vi "labviewFunc.vi"() -> ()   [LabVIEW 2022 SP3]
uses:
  <vilib>/DAQmx/write.llb/DAQmx Write (Analog DBL 1Chan 1Samp).vi
  <vilib>/DAQmx/read.llb/DAQmx Read (Analog DBL 1Chan 1Samp).vi
  <vilib>/DAQmx/read.llb/DAQmx Read (Counter 1D DBL 1Chan NSamp).vi
  <vilib>/Analysis/baseanly.llb/Mean (DBL).vi
  <vilib>/Utility/error.llb/Trim Whitespace One-Sided.vi
  <vilib>/Utility/file.llb/Read Delimited Spreadsheet (DBL).vi
  <vilib>/Utility/config.llb/Read Key (I32).vi
  <vilib>/Utility/config.llb/Read Key (String).vi
  <vilib>/DAQmx/create/channels.llb/DAQmx Create Channel (CI-Frequency).vi
  <vilib>/DAQmx/configure/timing.llb/DAQmx Timing (Implicit).vi
  <vilib>/DAQmx/create/channels.llb/DAQmx Create Channel (AO-Voltage-Basic).vi
  <vilib>/DAQmx/create/channels.llb/DAQmx Create Channel (AI-Voltage-Basic).vi
  <vilib>/DAQmx/miscellaneous.llb/DAQmx Fill In Error Info.vi
  <resource>/objmgr/daqmx.rc
  <vilib>/Analysis/NI_AALBase.lvlib
  <vilib>/Utility/config.llb/NI_LVConfig.lvlib
  <vilib>/Utility/config.llb/Read Key (Double).vi
panel:
  out "value 4":string
  out "all rows":dbl[](array[numeric])
  out "value 3":string
  out "value 2":string
  out "value":string
  in  "OK Button continue":bool
  in  "OK Button":bool
  out "fvar":variant
  out "ivar":variant
  out "ledVout":dbl[](array[numeric])
  in  "AIChannel":tag
  out "FreqOut":dbl[](array[numeric])
  in  "Delay":u32
  out "error out":errorcluster
  in  "AOChannel":tag
  in  "CounterPFI":tag
  in  "Counter":tag="Dev2/ctr0"
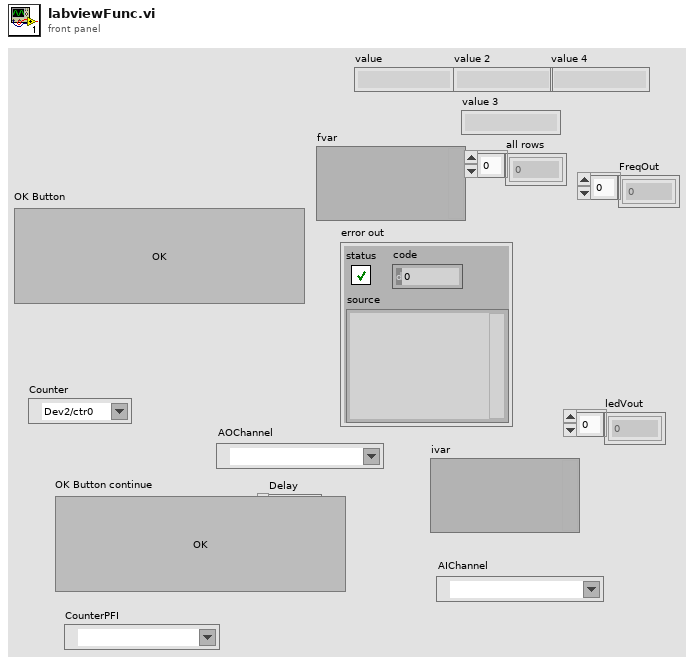
[diagram p1: front panel]
types:
  T1 = enum32{"Invalid", "Standard", "Closed", "Hidden", "Minimized", "Maximized"}
  T2 = typedef "NI_LVConfig.lvlib/Config Data RefNum.ctl" = refnum<k1>
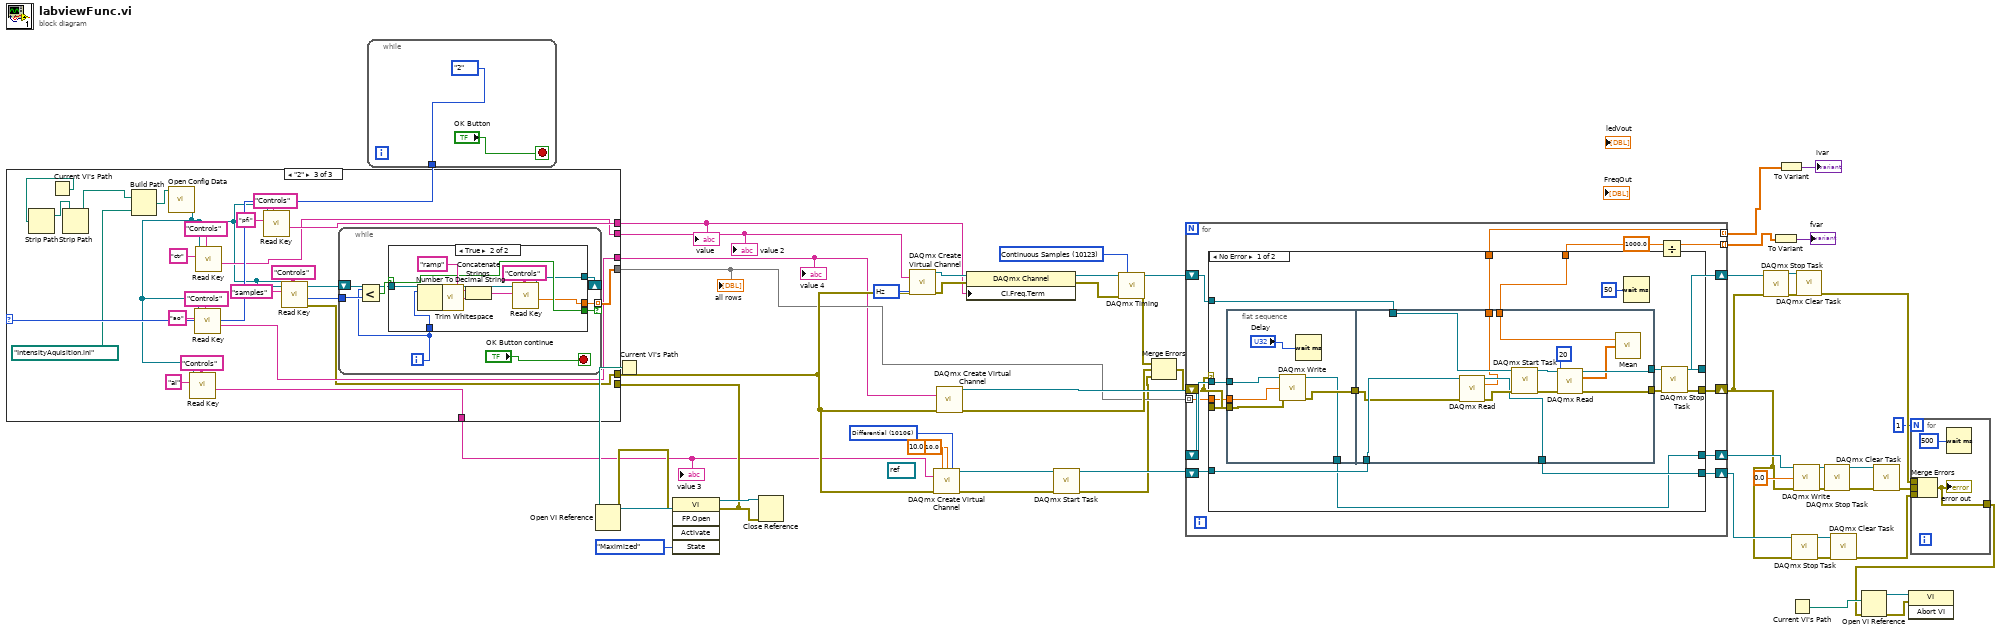
[diagram p0: block diagram]
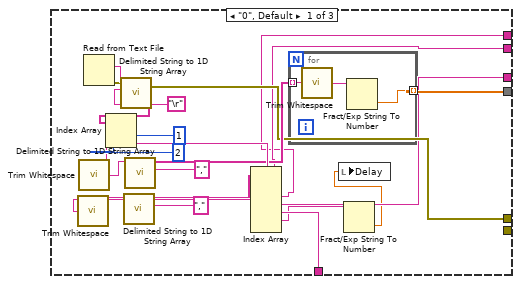
[diagram p2: hidden frame]
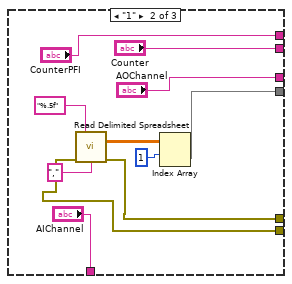
[diagram p3: hidden frame]
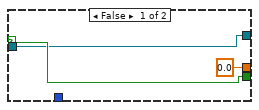
[diagram p4: hidden frame]
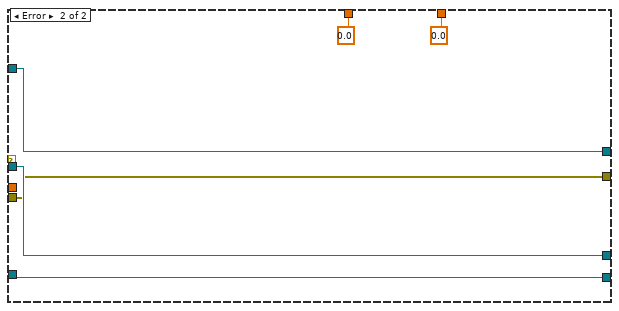
[diagram p5: hidden frame]
diagram:
  w28 = 10106 items=["Default"=-1, "RSE"=10083, "NRSE"=10078, "Differential"=10106, "Pseudodifferential"=12529] ("input terminal configuration")
  (unwired) refnum<k21> refnum ("task out")
  w42 = 10123 items=["Finite Samples"=10178, "Continuous Samples"=10123, "Hardware Timed Single Point"=12522] ("sample mode")
  w45 = 10373 items=["Hz"=10373, "Ticks"=10304, "From Custom Scale"=10065] ("units")
  n1 = while {
    tunnel: [enum16{"0", "1", "2"}."2"] -> w1
    stop <- "OK Button" stop-if-true
  }
  n2 = Current VI's Path() -> (path=w17:path)
  n3 = Open VI Reference(vi path=w17) -> (vi reference=w51:refnum<vi>, error out=w49:errorcluster)  [unwired: 5 in]
  n4 = invoke class="VI" method="FP.Open"(reference=w51, error in=w49, "State"=T1."Maximized") -> (reference out=w48:refnum<vi>, error out=w16:errorcluster)  [unwired: 2 in, 3 out]
  n5 = case shown="\"2\"" w1 {
    tunnel: w16 -> [_ w93 _]
    tunnel: [w67 w91 w101] -> w15
    tunnel: [w68 w89 w109] -> w14
    tunnel: [w65 "Counter" w107] -> w5
    tunnel: [w63 "AOChannel" w106] -> w4
    tunnel: [w62 "AIChannel" w105] -> w3
    tunnel: [w64 "CounterPFI" w108] -> w2
    frame "0", Default {
      n6 = Read from Text File() -> (text=w78:string, error out=w67:errorcluster)  [unwired: 4 in, 2 out]
      n7 = call <vilib>:"Delimited String to 1D String Array.vi"("delimiter"="\r", "delimited string"=w78) -> ("string array"=w77:string[])  [unwired: 9 in]
      n8 = Index Array(array=w77, index #1=1 ("index"), index #2=2 ("index")) -> (element #1=w74:string, element #2=w70:string)
      n9 = call <vilib>:"Trim Whitespace.vi"("string"=w70) -> ("trimmed string"=w59:string)  [unwired: 1 in]
      n10 = call <vilib>:"Trim Whitespace.vi"("string"=w74) -> ("trimmed string"=w73:string)  [unwired: 1 in]
      n11 = call <vilib>:"Delimited String to 1D String Array.vi"("delimiter"=",", "delimited string"=w59) -> ("string array"=w66:string[])  [unwired: 9 in]
      n12 = call <vilib>:"Delimited String to 1D String Array.vi"("delimiter"=",", "delimited string"=w73) -> ("string array"=w69:string[])  [unwired: 9 in]
      n13 = Index Array(array=w66) -> (element #1=w65:string, element #2=w64:string, element #3=w63:string, element #4=w62:string, element #5=w61:string)  [unwired: 6 in, 1 out]
      n14 = for {
        tunnel: w69 -> [w82] mode=indexing
        tunnel: [w80] -> w68 mode=indexing
        n15 = call <vilib>:"Trim Whitespace.vi"("string"=w82) -> ("trimmed string"=w81:string)  [unwired: 1 in]
        n16 = Fract/Exp String To Number(string=w81) -> (number=w80:dbl)  [unwired: 3 in, 1 out]
      }
      n17 = Fract/Exp String To Number(string=w61) -> (number=w60:dbl)  [unwired: 3 in, 1 out]
      n18 = local write "Delay"(w60) -> ()
    }
    frame "1" {
      n19 = call-poly <vilib>:"Read Delimited Spreadsheet.vi"("format (%.3f)"="%.5f", "error in (no error)"=w93, "delimiter (\\t)"="," ("delimiter (\\t)")) -> ("all rows"=w88:dbl[][], "error out"=w91:errorcluster)  [unwired: 7 in, 4 out]
      n20 = Index Array(array=w88, index (row)=1 ("index")) -> (element=w89:dbl[])  [unwired: 1 in]
    }
    frame "2" {
      n21 = Current VI's Path() -> (path=w98:path)
      n22 = Strip Path(path=w98) -> (stripped path=w97:path)  [unwired: 1 out]
      n23 = Strip Path(path=w97) -> (stripped path=w95:path)  [unwired: 1 out]
      n24 = Build Path(base path=w95, name or relative path=path "IntensityAquisition.ini") -> (appended path=w96:path)
      n25 = call <vilib>:"Open Config Data.vi"("configuration file path"=w96) -> ("refnum"=w103:T2)  [unwired: 8 in, 2 out]
      n26 = call-poly <vilib>:"Read Key.vi"("section"="Controls", "key"="ai", "refnum"=w103) -> ("value"=w105:string)  [unwired: 5 in, 3 out]
      n27 = call-poly <vilib>:"Read Key.vi"("section"="Controls", "key"="ao", "refnum"=w103) -> ("value"=w106:string)  [unwired: 5 in, 3 out]
      n28 = call-poly <vilib>:"Read Key.vi"("section"="Controls", "key"="ctr", "refnum"=w103) -> ("value"=w107:string)  [unwired: 5 in, 3 out]
      n29 = call-poly <vilib>:"Read Key.vi"("section"="Controls", "key"="pfi", "refnum"=w103) -> ("value"=w108:string)  [unwired: 5 in, 3 out]
      n30 = call-poly <vilib>:"Read Key.vi"("section"="Controls", "key"="samples", "refnum"=w103) -> ("error out"=w101:errorcluster, "value"=w104:i32)  [unwired: 5 in, 2 out]
      n31 = while {
        tunnel: [w124] -> w109 mode=indexing if=w121
        tunnel: w104 -> [w118]
        shift-right: [w119] -> _
        shift-left: w103 -> [w120]
        i -> [w117]
        stop <- "OK Button continue" stop-if-true
        n32 = Less?(x=w117, y=w118) -> (x < y?=w122:bool)
        n33 = case shown="True" w122 {
          selector: w122 -> [w126 w133]
          tunnel: w117 -> [_ w137]
          tunnel: [0.0 w129] -> w124
          tunnel: [w126 w133] -> w121
          tunnel: w120 -> [w125 w132]
          tunnel: [w125 w131] -> w119
          frame False {
          }
          frame True {
            n34 = Number To Decimal String(number=w137) -> (decimal integer string=w136:string)  [unwired: 1 in]
            n35 = call <vilib>:"Trim Whitespace.vi"("string"=w136) -> ("trimmed string"=w128:string)  [unwired: 1 in]
            n36 = Concatenate Strings("ramp" ("string"), w128) -> (w134:string)
            n37 = call-poly <vilib>:"Read Key.vi"("section"="Controls", "key"=w134, "refnum"=w132) -> ("value"=w129:dbl, "refnum out"=w131:T2)  [unwired: 5 in, 2 out]
          }
        }
      }
    }
  }
  "value" <- w2
  "value 2" <- w5
  "value 3" <- w3
  "all rows" <- w14
  "value 4" <- w4
  n38 = Close Reference(reference=w48, error in (no error)=w16) -> ()  [unwired: 1 out]
  n39 = call-poly <vilib>:"DAQmx Create Virtual Channel.vi"("counter"=w5, "units"=w45, "error in"=w15) -> ("task out"=w47:refnum<k21>, "error out"=w46:errorcluster)  [unwired: 11 in]
  n40 = call-poly <vilib>:"DAQmx Create Virtual Channel.vi"("maximum value"=10.0, "minimum value"=-10.0, "input terminal configuration"=w28, "physical channels"=w3, "error in"=w15) -> ("task out"=w13:refnum<k21>, "error out"=w11:errorcluster)  [unwired: 9 in]
  n41 = call-poly <vilib>:"DAQmx Create Virtual Channel.vi"("physical channels"=w4, "error in"=w15) -> ("task out"=w40:refnum<k21>, "error out"=w36:errorcluster)  [unwired: 12 in]
  n42 = property class="DAQmx Channel"(reference=w47, error in=w46, "CI.Freq.Term"=w2) -> (reference out=w44:refnum<k21>, error out=w43:errorcluster)
  n43 = call <vilib>:"DAQmx Start Task.vi"("task/channels in"=w13, "error in"=w11) -> ("task out"=w12:refnum<k21>, "error out"=w10:errorcluster)  [unwired: 12 in]
  n44 = call-poly <vilib>:"DAQmx Timing.vi"("task/channels in"=w44, "sample mode"=w42, "error in"=w43) -> ("task out"=w38:refnum<k21>, "error out"=w37:errorcluster)  [unwired: 11 in]
  n45 = Merge Errors(w37, w36, w10) -> (w35:errorcluster)
  n46 = for {
    tunnel: w14 -> [w149] mode=indexing
    shift-right: [w148] -> w39
    shift-left: w40 -> [w150]
    shift-right: [w146] -> w34
    shift-left: w38 -> [w147]
    shift-right: [w145] -> w24
    shift-left: w35 -> [w144]
    tunnel: [w139] -> w6 mode=indexing
    shift-right: [w141] -> w25
    shift-left: w12 -> [w142]
    tunnel: [w140] -> w9 mode=indexing
    n47 = case shown="No Error" w144 {
      tunnel: w150 -> [w164 w189]
      tunnel: w149 -> [w163 _]
      tunnel: [w155 w189] -> w148
      tunnel: w147 -> [w162 w190]
      tunnel: [w153 w190] -> w146
      tunnel: w144 -> [w160 w188]
      tunnel: [w151 w188] -> w145
      tunnel: [w159 0.0 ("mean")] -> w143
      tunnel: w142 -> [w158 w186]
      tunnel: [w157 w186] -> w141
      tunnel: [w156 0.0 ("data")] -> w140
      frame No Error {
        n48 = flat-sequence {
          tunnel: w164 -> [w171]
          tunnel: w163 -> [w166]
          tunnel: w160 -> [w169]
          tunnel: [w168] -> w165
          tunnel: [w167] -> w155
          tunnel: w162 -> [w177]
          tunnel: [w183] -> w161
          tunnel: [w182] -> w152
          tunnel: w165 -> [w174]
          tunnel: [w180] -> w159
          tunnel: w158 -> [w175]
          tunnel: [w173] -> w157
          tunnel: [w172] -> w156
          frame #0 {
            n49 = call-poly <vilib>:"DAQmx Write.vi"("task/channels in"=w171, "data"=w166, "error in"=w169) -> ("task out"=w167:refnum<k21>, "error out"=w168:errorcluster)  [unwired: 10 in, 1 out]
            n50 = Wait (ms)(milliseconds to wait="Delay") -> ()  [unwired: 1 out]
          }
          frame #1 {
            n51 = call-poly <vilib>:"DAQmx Read.vi"("task/channels in"=w175, "error in"=w174) -> ("task out"=w173:refnum<k21>, "data"=w172:dbl, "error out"=w176:errorcluster)  [unwired: 11 in]
            n52 = call <vilib>:"DAQmx Start Task.vi"("task/channels in"=w177, "error in"=w176) -> ("task out"=w179:refnum<k21>, "error out"=w178:errorcluster)  [unwired: 12 in]
            n53 = call-poly <vilib>:"DAQmx Read.vi"("task/channels in"=w179, "number of samples per channel"=20, "error in"=w178) -> ("task out"=w183:refnum<k21>, "data"=w181:dbl[], "error out"=w182:errorcluster)  [unwired: 10 in]
            n54 = call-poly <vilib>:"Mean.vi"("X"=w181) -> ("mean"=w180:dbl)  [unwired: 1 out]
          }
        }
        n55 = Wait (ms)(milliseconds to wait=u32 50) -> ()  [unwired: 1 out]
        n56 = call <vilib>:"DAQmx Stop Task.vi"("task/channels in"=w161, "error in"=w152) -> ("task out"=w153:refnum<k21>, "error out"=w151:errorcluster)  [unwired: 12 in]
      }
      frame Error {
      }
    }
    n57 = Divide(x=w143, y=1000.0) -> (x/y=w139:dbl)
  }
  n58 = call <vilib>:"DAQmx Stop Task.vi"("task/channels in"=w34, "error in"=w24) -> ("task out"=w33:refnum<k21>, "error out"=w32:errorcluster)  [unwired: 12 in]
  n59 = To Variant(anything=w6) -> (Variant=→"fvar":variant)
  n60 = To Variant(anything=w9) -> (Variant=→"ivar":variant)
  n61 = Current VI's Path() -> (path=w21:path)
  n62 = call <vilib>:"DAQmx Stop Task.vi"("task/channels in"=w25, "error in"=w24) -> ("task out"=w27:refnum<k21>, "error out"=w26:errorcluster)  [unwired: 12 in]
  n63 = call-poly <vilib>:"DAQmx Write.vi"("task/channels in"=w39, "data"=0.0, "error in"=w24) -> ("task out"=w53:refnum<k21>, "error out"=w54:errorcluster)  [unwired: 10 in, 1 out]
  n64 = call <vilib>:"DAQmx Clear Task.vi"("task in"=w33, "error in"=w32) -> ("error out"=w31:errorcluster)  [unwired: 13 in]
  n65 = call <vilib>:"DAQmx Stop Task.vi"("task/channels in"=w53, "error in"=w54) -> ("task out"=w56:refnum<k21>, "error out"=w55:errorcluster)  [unwired: 12 in]
  n66 = call <vilib>:"DAQmx Clear Task.vi"("task in"=w27, "error in"=w26) -> ("error out"=w23:errorcluster)  [unwired: 13 in]
  n67 = call <vilib>:"DAQmx Clear Task.vi"("task in"=w56, "error in"=w55) -> ("error out"=w41:errorcluster)  [unwired: 13 in]
  n68 = for {
    N: 1 -> [_]
    tunnel: w41 -> [w195]
    tunnel: w31 -> [w194]
    tunnel: w23 -> [w193]
    tunnel: [w191] -> w20
    n69 = Merge Errors(w194, w195, w193) -> (w191:errorcluster)
    "error out" <- w191
    n70 = Wait (ms)(milliseconds to wait=u32 500) -> ()  [unwired: 1 out]
  }
  n71 = Open VI Reference(vi path=w21, error in (no error)=w20) -> (vi reference=w19:refnum<vi>, error out=w18:errorcluster)  [unwired: 4 in]
  n72 = invoke class="VI" method="Abort VI"(reference=w19, error in=w18) -> ()  [unwired: 1 in, 3 out]
